vi "XML to Persistent Data.vi"(0 "XML Data":string) -> ()   [LabVIEW 2013]
uses:
  Types/Persistent Data.ctl
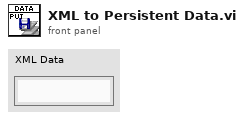
[diagram p1: front panel]
types:
  T1 = typedef "Persistent Data.ctl" = cluster{"File Name":string, "Save Directory":path, "Version":string}
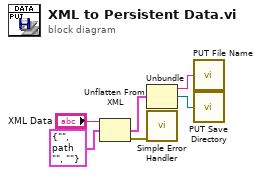
[diagram p0: block diagram]
diagram:
  n1 = Unflatten From XML(xml string="XML Data", type=T1 {"File Name"="", "Save Directory"=path "", "Version"=""} ("Persistent Data")) -> (value=w3:T1, error out=w6:errorcluster)  [unwired: 1 in]
  n2 = Unbundle(w3) -> ("File Name"=w2:string, "Save Directory"=w1:path)  [unwired: 1 out]
  n3 = call <vilib>:"Simple Error Handler.vi"("error in (no error)"=w6) -> ()  [unwired: 4 in, 5 out]
  n4 = call "PUT File Name.vi"("File Name"=w2) -> ()
  n5 = call "PUT Save Directory.vi"("Save Directory"=w1) -> ()
